vi "DashboardMain.vi"() -> ()   [LabVIEW 2014]
uses:
  RobotToDashboardCluster.ctl
  DashboardToRobotCluster.ctl
panel:
  out "Image":T1(plugin-control)
  out "Air Pressure":dbl(slide) scale=0.0..100.0
  out "Heading":dbl(knob) scale=0.0..360.0
  out "Attempting to Connect":bool
  out "Connected":bool
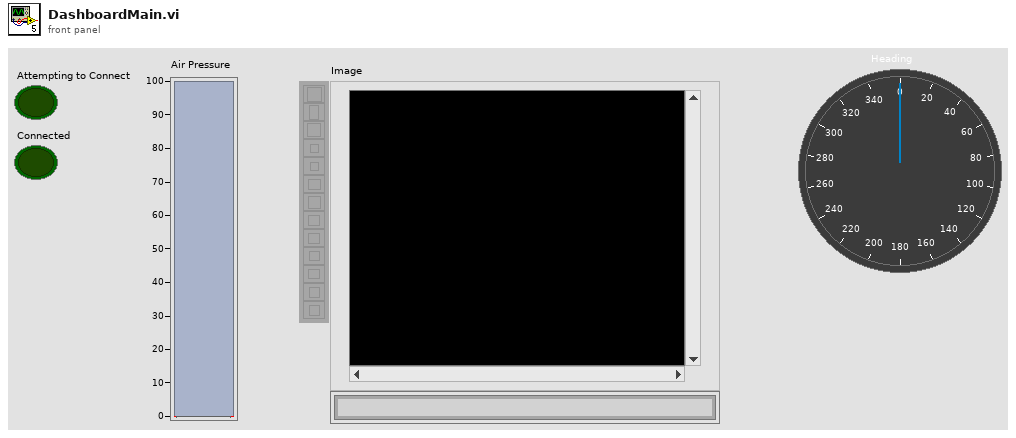
[diagram p1: front panel]
types:
  T1 = typedef "IMAQ Image.ctl" = refnum<image>
  T2 = typedef "DashboardToRobotCluster.ctl" = cluster{"Test":dbl}
  T3 = typedef "RobotToDashboardCluster.ctl" = cluster{"Front Right Motor":dbl, "Front Left Motor":dbl, "Rear Right Motor":dbl, "Rear Left Motor":dbl, "Current Heading":dbl, "Can Grabber Closed":bool, "Tote lift Up":bool, "Feeders Running":bool, "Pressure In Tank":dbl, "Image String":string}
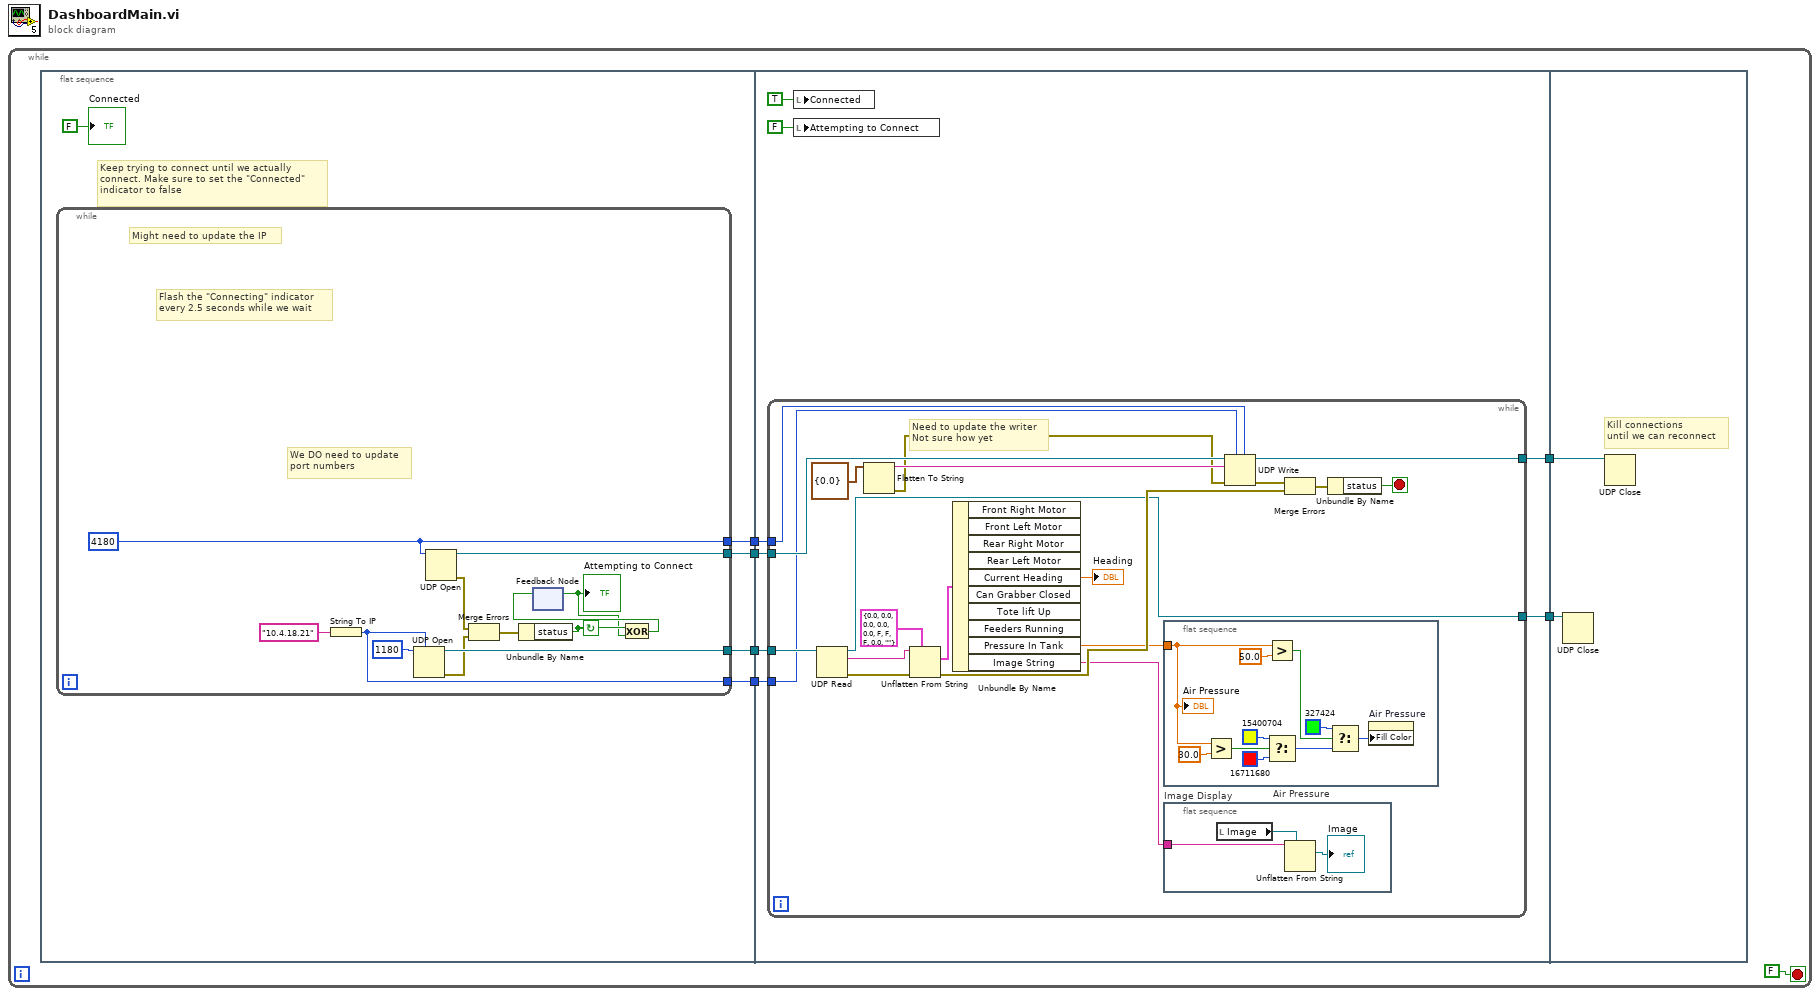
[diagram p0: block diagram]
diagram:
  n1 = while {
    stop <- FALSE stop-if-true
    n2 = flat-sequence {
      tunnel: [w12] -> w6
      tunnel: [w11] -> w5
      tunnel: [w10] -> w4
      tunnel: [w9] -> w3
      tunnel: w6 -> [w32]
      tunnel: w5 -> [w30]
      tunnel: w4 -> [w29]
      tunnel: w3 -> [w28]
      tunnel: [w26] -> w2
      tunnel: [w25] -> w1
      tunnel: w2 -> [w67]
      tunnel: w1 -> [w66]
      frame #0 {
        # "Keep trying to connect until we actually\nconnect. Make sure to set the \"Connected\"\nindicator to false"
        n3 = while {
          tunnel: [w20] -> w12
          tunnel: [w16] -> w11
          tunnel: [w15] -> w10
          tunnel: [w14] -> w9
          stop <- w21 continue-if-true
          w14 = u16 4180 ("port")
          # "We DO need to update\nport numbers"
          # "Might need to update the IP"
          # "Flash the \"Connecting\" indicator\nevery 2.5 seconds while we wait"
          n4 = String To IP(1:"10.4.18.21" ("name")) -> (0:w15:u32)
          n5 = UDP Open(7:w15, 11:u16 1180 ("port")) -> (port=w20:refnum<k16>, 0:w18:errorcluster)  [unwired: 3 in, 1 out]
          n6 = UDP Open(11:w14) -> (port=w16:refnum<k16>, 0:w19:errorcluster)  [unwired: 4 in, 1 out]
          n7 = Merge Errors(w19, w18) -> (w17:errorcluster)
          n8 = Unbundle By Name(w17) -> ("status"=w21:bool)
          n9 = feedback #1() -> (w13:bool)  [unwired: 1 in]
          "Attempting to Connect" <- w13
          n10 = Exclusive Or(1:w13, 2:w21) -> (0:w22:bool)
          n11 = feedback-in #1(w22) -> ()
        }
        "Connected" <- FALSE ("Communications")
      }
      frame #1 {
        n12 = while {
          tunnel: w32 -> [w47]
          tunnel: w30 -> [w46]
          tunnel: w29 -> [w45]
          tunnel: w28 -> [w44]
          tunnel: [w38] -> w26
          tunnel: [w37] -> w25
          stop <- w50 stop-if-true
          # "Need to update the writer\nNot sure how yet"
          n13 = UDP Read(connection ID=w47) -> (data out=w52:string, error out=w51:errorcluster, 3:w37:refnum<k16>)  [unwired: 3 in, 2 out]
          n14 = Flatten To String(anything=T2 {"Test"=0.0} ("Cluster")) -> (data string=w43:string, error out=w42:errorcluster)  [unwired: 3 in, 1 out]
          n15 = Unflatten From String(type=T3 {"Front Right Motor"=0.0, "Front Left Motor"=0.0, "Rear Right Motor"=0.0, "Rear Left Motor"=0.0, "Current Heading"=0.0, "Can Grabber Closed"=FALSE, "Tote lift Up"=FALSE, "Feeders Running"=FALSE, "Pressure In Tank"=0.0, "Image String"=""} ("Dashboard Cluster"), binary string=w52, error in (no error)=w51) -> (value=w48:T3, error out=w40:errorcluster)  [unwired: 2 in, 1 out]
          n16 = Unbundle By Name(w48) -> ("Current Heading"=→"Heading":dbl, "Pressure In Tank"=w34:dbl, "Image String"=w33:string)  [unwired: 7 out]
          n17 = flat-sequence "Air Pressure" {
            tunnel: w34 -> [w58]
            frame #0 {
              n18 = Greater?(x=w58, y=30.0) -> (0:w59:bool)
              n19 = Greater?(x=w58, y=50.0) -> (0:w64:bool)
              n20 = Select(t=u32 15400704, s=w59, f=u32 16711680) -> (s? t:f=w61:u32)
              n21 = Select(t=u32 327424, s=w64, f=w61) -> (s? t:f=w62:u32)
              n22 = property on="Air Pressure" class="Slide (strict)"("Fill Color"=w62) -> ()  [unwired: 2 in, 2 out]
              "Air Pressure" <- w58
            }
          }
          n23 = flat-sequence "Image Display" {
            tunnel: w33 -> [w55]
            frame #0 {
              n24 = local read "Image"() -> (w54:T1)
              n25 = Unflatten From String(type=w54, binary string=w55) -> (value=→"Image":T1)  [unwired: 3 in, 2 out]
            }
          }
          n26 = UDP Write(address=w45, port or service name=w44, connection ID=w46, data in=w43, 8:w42) -> (error out=w41:errorcluster, 3:w38:refnum<k16>)  [unwired: 1 in]
          n27 = Merge Errors(w41, w40) -> (w39:errorcluster)
          n28 = Unbundle By Name(w39) -> ("status"=w50:bool)
        }
        n29 = local write "Connected"(TRUE ("Connected")) -> ()
        n30 = local write "Attempting to Connect"(FALSE ("Connecting")) -> ()
      }
      frame #2 {
        # "Kill connections\nuntil we can reconnect"
        n31 = UDP Close(connection ID=w66) -> ()  [unwired: 1 in, 2 out]
        n32 = UDP Close(connection ID=w67) -> ()  [unwired: 1 in, 2 out]
      }
    }
  }
